vi "Excel Stat Division Lines.vi"(8 "Error In":errorcluster, 10 "Data In":string[][](array[string]), 11 "Cells Ref In":refnum<k7>) -> (0 "Error Out":errorcluster, 3 "Cells Ref Out":refnum<k7>)   [LabVIEW 2013]
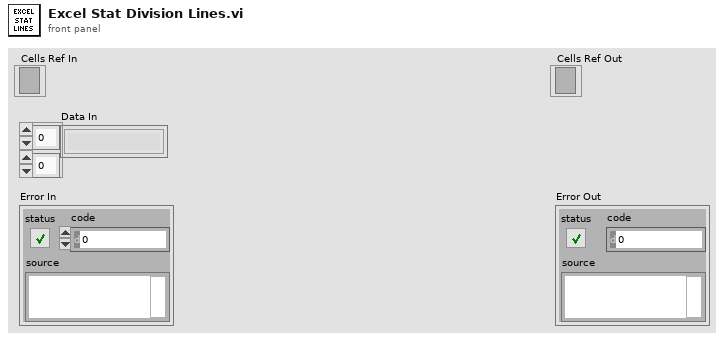
[diagram p1: front panel]
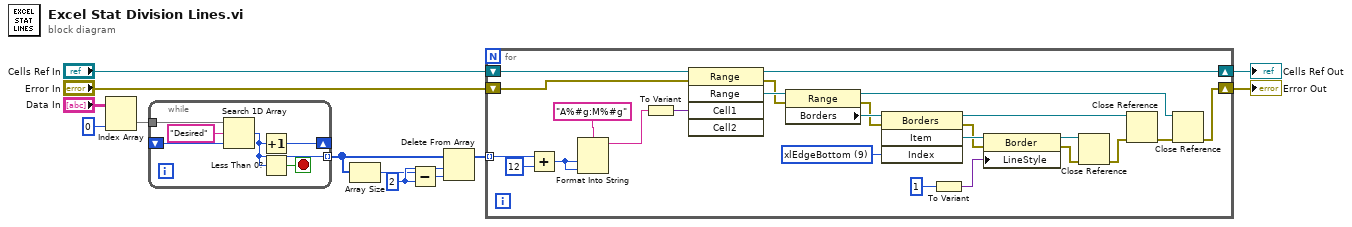
[diagram p0: block diagram]
diagram:
  w10 = 2 ("y")
  n1 = Index Array(array="Data In", index (col)=0 ("disabled index (col)")) -> (element=w7:string[])  [unwired: 1 in]
  n2 = while {
    tunnel: w7 -> [w18]
    shift-right: [w15] -> _
    shift-left: _ -> [w16]
    tunnel: [w14] -> w11 mode=indexing
    stop <- w13 stop-if-true
    n3 = Search 1D Array(1D array=w18, element="Desired", start index (0)=w16) -> (index of element=w14:i32)
    n4 = Increment(x=w14) -> (x+1=w15:i32)
    n5 = Less Than 0?(x=w14) -> (x < 0?=w13:bool)
  }
  n6 = Array Size(array=w11) -> (size(s)=w8:i32)
  n7 = Subtract(x=w8, y=w10) -> (x-y=w9:i32)
  n8 = Delete From Array(array=w11, length=w10, index=w9) -> (array with subset deleted=w12:i32[])  [unwired: 1 out]
  n9 = for {
    tunnel: w12 -> [w26] mode=indexing
    shift-right: [w22] -> w4
    shift-left: "Cells Ref In" -> [w23]
    shift-right: [w21] -> w3
    shift-left: "Error In" -> [w20]
    w27 = 9 items=["xlInsideHorizontal"=12, "xlInsideVertical"=11, "xlDiagonalDown"=5, "xlDiagonalUp"=6, "xlEdgeBottom"=9, "xlEdgeLeft"=7, "xlEdgeRight"=10, "xlEdgeTop"=8] ("Index")
    n10 = Add(x=w26, y=12) -> (x+y=w25:i32)
    n11 = Format Into String(format string="A%#g:M%#g", w25, w25) -> (resulting string=w19:string)  [unwired: 2 in, 1 out]
    n12 = To Variant(anything=w19) -> (Variant=w38:variant)
    n13 = invoke class="Range" method="Range"(reference=w23, error in=w20, "Cell1"=w38) -> (reference out=w22:refnum<k7>, error out=w41:errorcluster, "Range"=w43:refnum<k7>)  [unwired: 2 in, 2 out]
    n14 = property class="Range"(reference=w43, error in=w41) -> (reference out=w39:refnum<k7>, error out=w33:errorcluster, "Borders"=w35:refnum<k7>)
    n15 = invoke class="Borders" method="Item"(reference=w35, error in=w33, "Index"=w27) -> (reference out=w31:refnum<k7>, error out=w32:errorcluster, "Item"=w34:refnum<k7>)  [unwired: 1 in, 1 out]
    n16 = To Variant(anything=1 ("input 1")) -> (Variant=w37:variant)
    n17 = property class="Border"(reference=w34, error in=w32, "LineStyle"=w37) -> (reference out=w30:refnum<k7>, error out=w29:errorcluster)
    n18 = Close Reference(reference=w30, error in (no error)=w29) -> (error out=w28:errorcluster)
    n19 = Close Reference(reference=w31, error in (no error)=w28) -> (error out=w40:errorcluster)
    n20 = Close Reference(reference=w39, error in (no error)=w40) -> (error out=w21:errorcluster)
  }
  "Cells Ref Out" <- w4
  "Error Out" <- w3
